vi "Parse Event and log.vi"(8 "error in":errorcluster, 10 "Variant":variant, 11 "Report in":refnum<class "Report.lvclass">) -> (0 "error out":errorcluster, 3 "Report out":refnum<class "Report.lvclass">)   [LabVIEW 2023, in "Report.lvlib" / "Report.lvclass"]
uses:
  Report.lvclass
  Custom Controls/Event Data.ctl
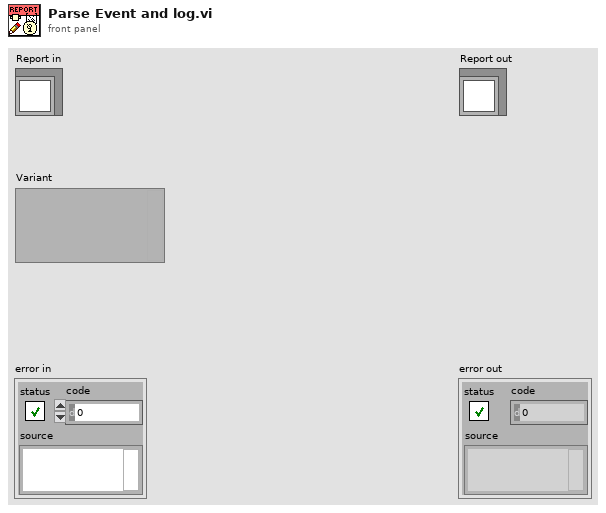
[diagram p1: front panel]
types:
  T1 = typedef "Report.lvlib/Report.lvclass/Event Data.ctl" = cluster{"Time Stamp":timestamp, "Instrument":string, "Description":string, "Data":string}
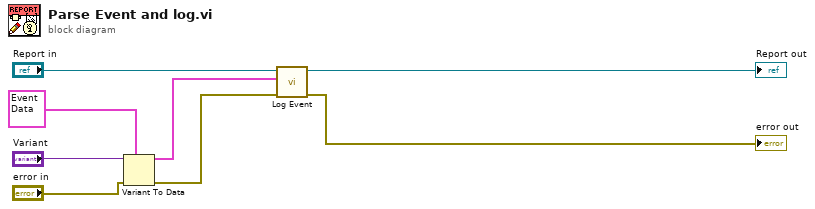
[diagram p0: block diagram]
diagram:
  n1 = Variant To Data(error in="error in", type=T1 {"Time Stamp"=timestamp(0 s since 1904-01-01), "Instrument"="", "Description"="", "Data"=""} ("Event Data"), Variant="Variant") -> (data=w1:T1, error out=w5:errorcluster)
  n2 = call-dynamic "Log Event.vi"("error in"=w5, "Event Data"=w1, "Report in"="Report in") -> ("error out"=→"error out":errorcluster, "Report out"=→"Report out":refnum<class "Report.lvclass">)  [unwired: 7 in]
